vi "Example - Manual Control.vi"() -> ()   [LabVIEW 2009, in "Digikrom DK24x.lvlib"]
doc: "Application example."
uses:
  Digikrom DK24x.lvlib
panel:
  in  "VISA resource name":refnum<visa-resource-name>="COM1"
  in  "DK24x Control Panel":T1={"Wavelength"=5.000000000000001e-07, "Slit 1 width"=1.0000000000000004e-05, "Slit 2 width"=1.0000000000000004e-05, "Filter"=1, "Grating"=1, "Ready"=FALSE} {"Grating" items=["250 nm"=1, "500 nm"=2, "2500 nm"=3]; "Filter" items=["No filter"=1, "345"=2, "550"=3, "1000"=4, "1500"=5, "2500"=6]; "Slit 2 width" min=1.0000000000000004e-05 max=0.005000000000000002 step=1.0000000000000004e-05; "Slit 1 width" min=1.0000000000000004e-05 max=0.005000000000000002 step=1.0000000000000004e-05; "Wavelength" min=0.0 max=6e-06 step=1.0000000000000008e-13 format="%.2f"}
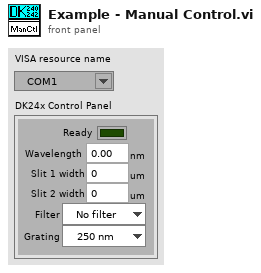
[diagram p1: front panel]
types:
  T1 = cluster{"Wavelength":dbl[unit], "Slit 1 width":dbl[unit], "Slit 2 width":dbl[unit], "Filter":u8, "Grating":u8, "Ready":bool}
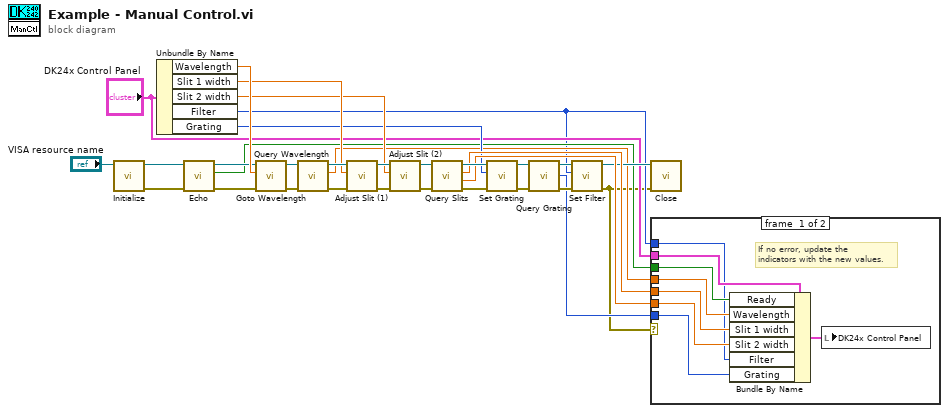
[diagram p0: block diagram]
diagram:
  n1 = call "Initialize.vi"("VISA resource name"="VISA resource name") -> ("error out"=w7:errorcluster, "VISA resource name out"=w8:refnum<visa-resource-name>)  [unwired: 3 in, 6 out]
  n2 = Unbundle By Name("DK24x Control Panel") -> ("Wavelength"=w16:dbl[unit], "Slit 1 width"=w15:dbl[unit], "Slit 2 width"=w14:dbl[unit], "Filter"=w4:u8, "Grating"=w13:u8)
  n3 = call "Echo.vi"("error in (no error)"=w7, "VISA resource name"=w8) -> ("error out"=w10:errorcluster, "Comm OK?"=w6:bool, "VISA resource name out"=w9:refnum<visa-resource-name>)  [unwired: 7 out]
  n4 = call "Goto Wavelength.vi"("error in (no error)"=w10, "WAVELENGTH"=w16, "VISA resource name"=w9) -> ("error out"=w30:errorcluster, "VISA resource name out"=w29:refnum<visa-resource-name>)  [unwired: 7 out]
  n5 = call "Query Wavelength.vi"("error in (no error)"=w30, "VISA resource name"=w29) -> ("error out"=w23:errorcluster, "CURRENT WAVELENGTH"=w11:dbl[unit], "VISA resource name out"=w24:refnum<visa-resource-name>)  [unwired: 7 out]
  n6 = call "Adjust Slit (1).vi"("error in (no error)"=w23, "SLIT WIDTH"=w15, "VISA resource name"=w24) -> ("error out"=w26:errorcluster, "VISA resource name out"=w25:refnum<visa-resource-name>)  [unwired: 7 out]
  n7 = call "Adjust Slit (2).vi"("error in (no error)"=w26, "SLIT WIDTH"=w14, "VISA resource name"=w25) -> ("error out"=w31:errorcluster, "VISA resource name out"=w32:refnum<visa-resource-name>)  [unwired: 7 out]
  n8 = call "Query Slits.vi"("error in (no error)"=w31, "VISA resource name"=w32) -> ("error out"=w22:errorcluster, "CURRENT S2 WIDTH"=w17:dbl[unit], "CURRENT S1 WIDTH"=w18:dbl[unit], "VISA resource name out"=w21:refnum<visa-resource-name>)  [unwired: 6 out]
  n9 = call "Set Grating.vi"("error in (no error)"=w22, "NEW GRT?"=w13, "VISA resource name"=w21) -> ("error out"=w27:errorcluster, "VISA resource name out"=w28:refnum<visa-resource-name>)  [unwired: 7 out]
  n10 = call "Query Grating.vi"("error in (no error)"=w27, "VISA resource name"=w28) -> ("error out"=w20:errorcluster, "GRATING #"=w3:u8, "VISA resource name out"=w19:refnum<visa-resource-name>)  [unwired: 7 out]
  n11 = call "Set Filter.vi"("error in (no error)"=w20, "NEW FILTER"=w4, "VISA resource name"=w19) -> ("error out"=w2:errorcluster, "VISA resource name out"=w12:refnum<visa-resource-name>)  [unwired: 7 out]
  n12 = call "Close.vi"("error in (no error)"=w2, "VISA resource name"=w12) -> ()  [unwired: 10 out]
  n13 = case shown="No Error" w2 {
    tunnel: w18 -> [w40 _]
    tunnel: w17 -> [w39 _]
    tunnel: w11 -> [w37 _]
    tunnel: w6 -> [w36 _]
    tunnel: "DK24x Control Panel" -> [w35 _]
    tunnel: w4 -> [w34 _]
    tunnel: w3 -> [w33 _]
    frame #0 {
      # "If no error, update the\nindicators with the new values."
      n14 = Bundle By Name(cluster=w35, "Ready"=w36, "Wavelength"=w37, "Slit 1 width"=w40, "Slit 2 width"=w39, "Filter"=w34, "Grating"=w33) -> (w38:T1)
      n15 = local write "DK24x Control Panel"(w38) -> ()
    }
    frame #1 {
    }
  }
